vi "2 axis-Move.vi"(1 "error in (no error)":errorcluster, 2 "Deceleration":bool, 5 "RESET":bool, 6 "Accelaration":bool, 7 "B axis":i32, 8 "Stop":bool, 9 "A axis":i32, 10 "Comport":refnum<visa-resource-name>="COM4") -> (3 "A out":dbl, 4 "B out":dbl)   [LabVIEW 2023]
uses:
  <vilib>/Instr/_visa.llb/VISA Configure Serial Port (Instr).vi
  Holmarc/2 axis linear/GlobalValue.vi
panel:
  out "x-y 2":u32
  out "x-y":u32
  out "Process 3":u32
  out "Process 2":u32
  out "movement\ntime":u32
  out "First loop":u32
  # "COMPORT"
  # "To Move"
  # "Moved"
  # "Microns"
  # "Microns"
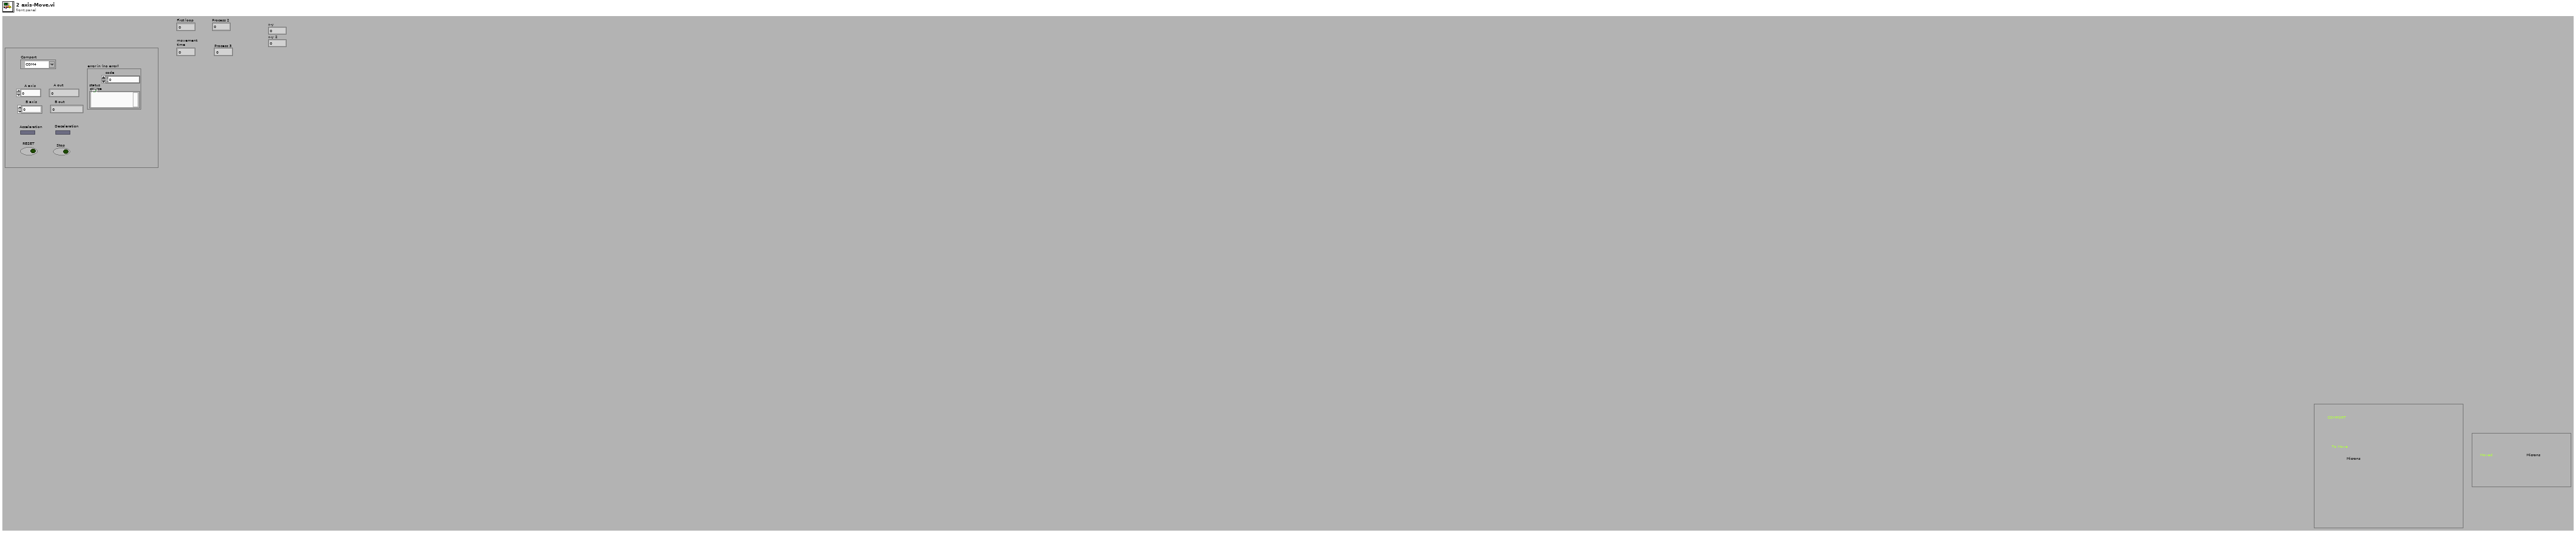
[diagram p1: front panel]
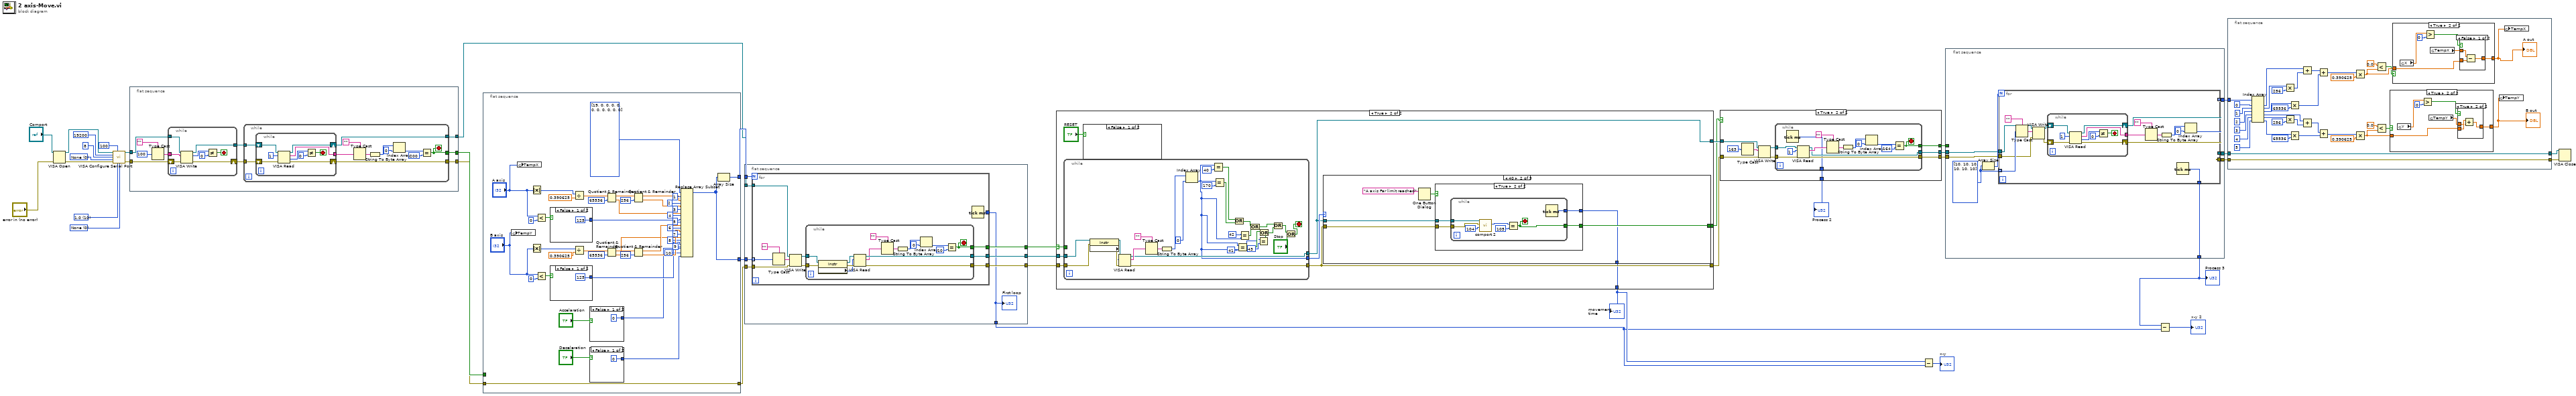
[diagram p0: block diagram]
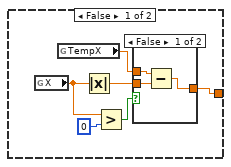
[diagram p2: hidden frame]
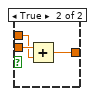
[diagram p3: hidden frame]
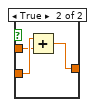
[diagram p4: hidden frame]
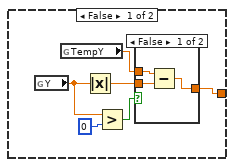
[diagram p5: hidden frame]
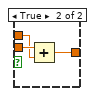
[diagram p6: hidden frame]
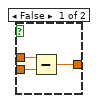
[diagram p7: hidden frame]
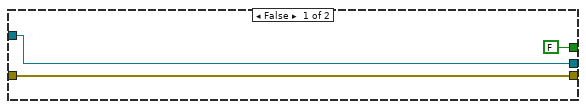
[diagram p8: hidden frame]
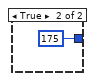
[diagram p9: hidden frame]
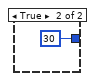
[diagram p10: hidden frame]
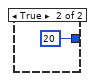
[diagram p11: hidden frame]
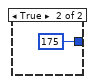
[diagram p12: hidden frame]
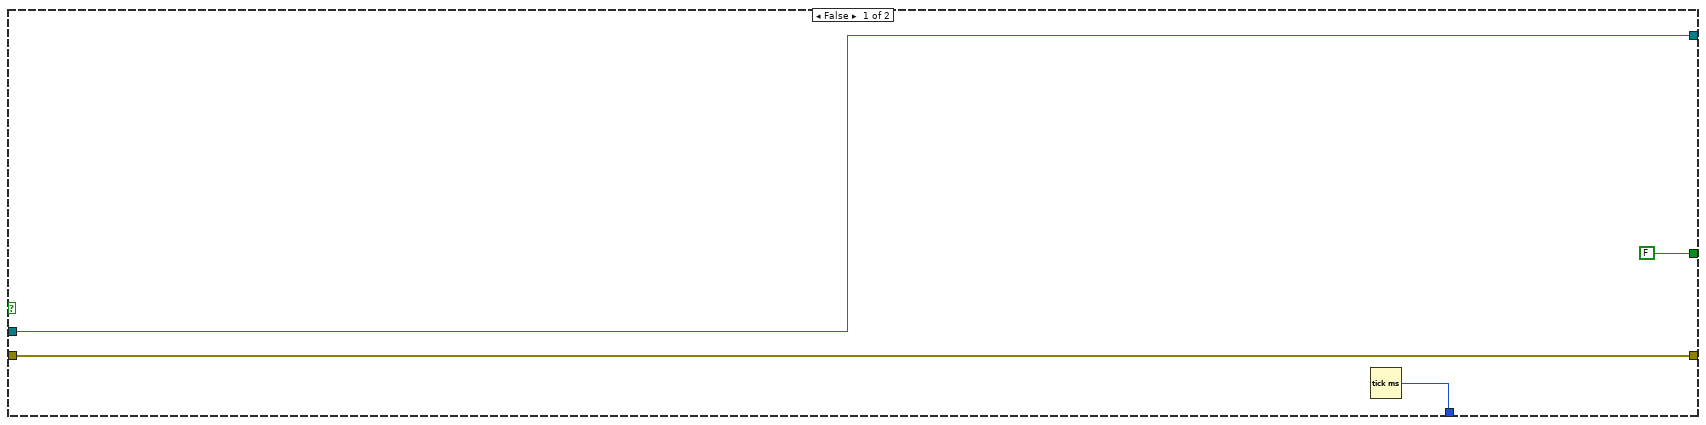
[diagram p13: hidden frame]
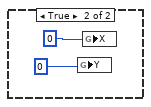
[diagram p14: hidden frame]
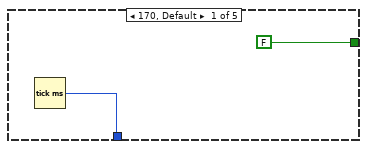
[diagram p15: hidden frame]
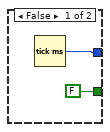
[diagram p16: hidden frame]
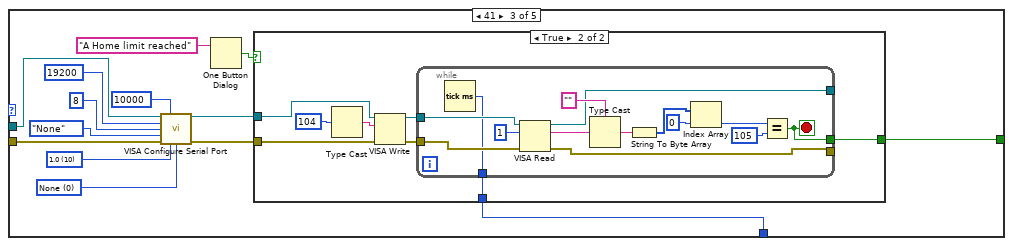
[diagram p17: hidden frame]
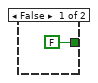
[diagram p18: hidden frame]
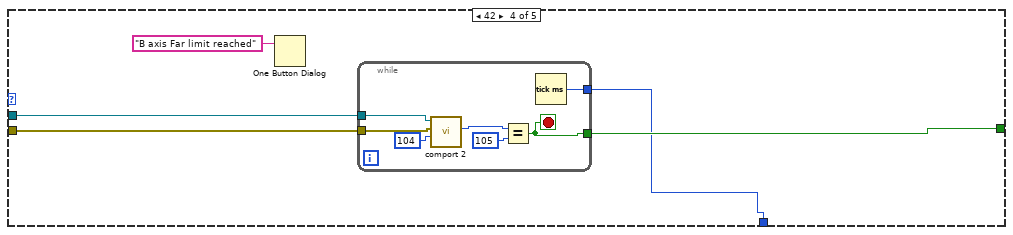
[diagram p19: hidden frame]
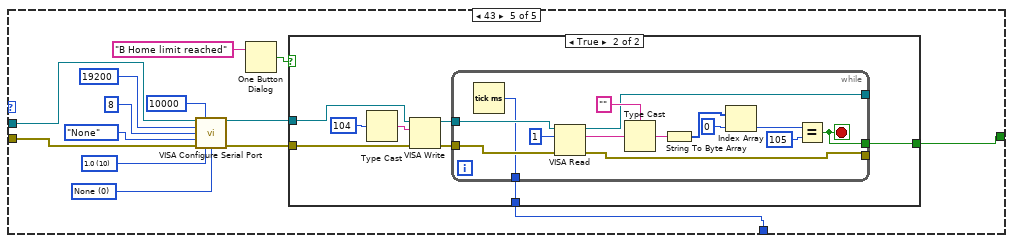
[diagram p20: hidden frame]
diagram:
  w33 = u16 0 items=["None"=0, "XON/XOFF"=1, "RTS/CTS"=2, "DTR/DSR"=4] ("flow control")
  w32 = u16 10 items=["1.0"=10, "1.5"=15, "2.0"=20] ("stop bits")
  w31 = u16 0 items=["None", "Odd", "Even", "Mark", "Space"] ("parity")
  n1 = VISA Open(error in (no error)="error in (no error)", VISA resource name="Comport") -> (VISA resource name=w36:refnum<visa-resource-name>, error out=w37:errorcluster)  [unwired: 3 in]
  n2 = call-poly "VISA Configure Serial Port"("VISA resource name"=w36, "timeout (10sec)"=u32 100, "baud rate (9600)"=u32 19200 ("baud rate"), "data bits (8)"=u16 8 ("data bits"), "parity (0:none)"=w31, "error in (no error)"=w37, "stop bits (10: 1 bit)"=w32, "flow control (0:none)"=w33) -> ("VISA resource name out"=w28:refnum<visa-resource-name>, "error out"=w27:errorcluster)  [unwired: 1 in, 5 out]
  n3 = flat-sequence {
    tunnel: w28 -> [w48]
    tunnel: w27 -> [w47]
    tunnel: [w46] -> w25
    tunnel: [w45] -> w12
    tunnel: [w39] -> w13
    frame #0 {
      n4 = Type Cast(type="", x=u8 100) -> (*(type *) &x=w43:string)
      n5 = while {
        tunnel: w43 -> [w56]
        shift-right: [w52] -> w40
        shift-left: w47 -> [w54]
        tunnel: w48 -> [w55]
        tunnel: [w53] -> w41
        stop <- w49 stop-if-true
        n6 = VISA Write(VISA resource name=w55, write buffer=w56, error in (no error)=w54) -> (VISA resource name out=w53:refnum<visa-resource-name>, return count=w51:u32, error out=w52:errorcluster)
        n7 = Not Equal?(x=w51, y=u32 0) -> (x != y?=w49:bool)
      }
      n8 = while {
        tunnel: w40 -> [w67]
        tunnel: [w65] -> w45
        tunnel: w41 -> [w68]
        tunnel: [w66] -> w46
        tunnel: [w60] -> w39
        stop <- w60 stop-if-true
        n9 = while {
          tunnel: [w72] -> w59
          shift-right: [w75] -> w66
          shift-left: w68 -> [w77]
          shift-right: [w74] -> w65
          shift-left: w67 -> [w76]
          stop <- w69 stop-if-true
          n10 = VISA Read(VISA resource name=w77, byte count=u32 1, error in (no error)=w76) -> (VISA resource name out=w75:refnum<visa-resource-name>, read buffer=w72:string, return count=w70:u32, error out=w74:errorcluster)
          n11 = Not Equal?(x=w70, y=u32 0) -> (x != y?=w69:bool)
        }
        n12 = Type Cast(type="", x=w59) -> (*(type *) &x=w57:string)
        n13 = String To Byte Array(string=w57) -> (unsigned byte array=w64:u8[])
        n14 = Index Array(array=w64, index=0) -> (element=w62:u8)
        n15 = Equal?(x=w62, y=u8 200) -> (x = y?=w60:bool)
      }
    }
  }
  n16 = flat-sequence {
    tunnel: [w116] -> w26
    tunnel: [w78] -> w24
    tunnel: w13 -> [_]
    tunnel: w12 -> [w113]
    tunnel: [w113] -> w11
    frame #0 {
      n17 = global write "GlobalValue.vi" "TempY"("B axis") -> ()
      n18 = global write "GlobalValue.vi" "TempX"("A axis") -> ()
      n19 = Absolute Value(x="A axis") -> (abs(x)=w117:i32)
      n20 = Absolute Value(x="B axis") -> (abs(x)=w105:i32)
      n21 = Less?(x="A axis", y=0) -> (x < y?=w119:bool)
      n22 = Less?(x="B axis", y=0) -> (x < y?=w100:bool)
      n23 = case shown="False" w119 {
        tunnel: [u16 125 u16 175] -> w91
        frame False {
        }
        frame True {
        }
      }
      n24 = case shown="False" w100 {
        tunnel: [u16 125 u16 175] -> w83
        frame False {
        }
        frame True {
        }
      }
      n25 = Divide(x=w117, y=0.390625) -> (x/y=w112:dbl)
      n26 = Divide(x=w105, y=0.390625) -> (x/y=w104:dbl)
      n27 = case shown="False" "Accelaration" {
        tunnel: [0 20] -> w81
        frame False {
        }
        frame True {
        }
      }
      n28 = case shown="False" "Deceleration" {
        tunnel: [0 30] -> w79
        frame False {
        }
        frame True {
        }
      }
      n29 = Quotient & Remainder(x=w112, y=65536) -> (x-y*floor(x/y)=w110:dbl, floor(x/y)=w94:dbl)
      n30 = Quotient & Remainder(x=w104, y=65536) -> (x-y*floor(x/y)=w102:dbl, floor(x/y)=w85:dbl)
      n31 = Quotient & Remainder(x=w110, y=256) -> (x-y*floor(x/y)=w97:dbl, floor(x/y)=w96:dbl)
      n32 = Quotient & Remainder(x=w102, y=256) -> (x-y*floor(x/y)=w89:dbl, floor(x/y)=w87:dbl)
      n33 = Replace Array Subset(array=u8[] [19, 0, 0, 0, 0, 0, 0, 0, 0, 0, 0], new element #1=w97, index #1=1 ("index"), new element #2=w96, index #2=2 ("index"), new element #3=w94, index #3=3 ("index"), new element #4=w91, index #4=4 ("index"), new element #5=w89, index #5=5 ("index"), new element #6=w87, index #6=6 ("index"), new element #7=w85, index #7=7 ("index"), new element #8=w83, index #8=8 ("index"), new element #9=w81, index #9=9 ("index"), new element #10=w79, index #10=10 ("index")) -> (w78:u8[])
      n34 = Array Size(array=w78) -> (size(s)=w116:i32)
    }
  }
  n35 = flat-sequence {
    tunnel: w26 -> [w137]
    tunnel: w25 -> [w136]
    tunnel: w11 -> [w135]
    tunnel: w24 -> [w134]
    tunnel: [w133] -> w23
    tunnel: [w132] -> w10
    tunnel: [w131] -> w22
    tunnel: [w130] -> w3
    frame #0 {
      n36 = for {
        N: w137 -> [_]
        tunnel: [w143] -> w131
        tunnel: w136 -> [w147]
        tunnel: [w145] -> w133
        tunnel: w135 -> [w146]
        tunnel: [w144] -> w132
        tunnel: w134 -> [w140] mode=indexing
        tunnel: [w138] -> w130
        n37 = Type Cast(type="", x=w140) -> (*(type *) &x=w139:string)
        n38 = VISA Write(VISA resource name=w147, write buffer=w139, error in (no error)=w146) -> (VISA resource name out=w142:refnum<visa-resource-name>, error out=w141:errorcluster)  [unwired: 1 out]
        n39 = while {
          tunnel: w141 -> [w152]
          tunnel: [w162] -> w144
          tunnel: w142 -> [w153]
          tunnel: [w163] -> w145
          tunnel: [w157] -> w143
          stop <- w157 stop-if-true
          n40 = property class="Instr"(reference=w153, error in=w152) -> (reference out=w151:refnum<visa-resource-name>, error out=w150:errorcluster, "Serial Settings:Number of Bytes at Serial Port"=w149:u32)
          n41 = VISA Read(VISA resource name=w151, byte count=w149, error in (no error)=w150) -> (VISA resource name out=w163:refnum<visa-resource-name>, read buffer=w156:string, error out=w162:errorcluster)  [unwired: 1 out]
          n42 = Type Cast(type="", x=w156) -> (*(type *) &x=w154:string)
          n43 = String To Byte Array(string=w154) -> (unsigned byte array=w161:u8[])
          n44 = Index Array(array=w161, index=0) -> (element=w159:u8)
          n45 = Equal?(x=w159, y=u8 10) -> (x = y?=w157:bool)
        }
        n46 = Tick Count (ms)() -> (millisecond timer value=w138:u32)
      }
      "First loop" <- w130
    }
  }
  n47 = case shown="True" w22 {
    selector: w22 -> [_ w169]
    tunnel: w23 -> [w167 w173]
    tunnel: w10 -> [w166 w175]
    tunnel: [w167 w172] -> w21
    tunnel: [w166 w171] -> w20
    tunnel: [FALSE w170] -> w7
    tunnel: [w164 w168] -> w5
    frame False {
      n48 = Tick Count (ms)() -> (millisecond timer value=w164:u32)
    }
    frame True {
      n49 = while {
        tunnel: w175 -> [w191]
        tunnel: [w195] -> w172
        tunnel: [w197] -> w171
        tunnel: [w177] -> w174
        tunnel: w173 -> [w192]
        tunnel: w169 -> [_]
        stop <- w178 stop-if-true
        n50 = property class="Instr"(reference=w192, error in=w191) -> (reference out=w190:refnum<visa-resource-name>, error out=w189:errorcluster, "Serial Settings:Number of Bytes at Serial Port"=w188:u32)
        n51 = VISA Read(VISA resource name=w190, byte count=w188, error in (no error)=w189) -> (VISA resource name out=w195:refnum<visa-resource-name>, read buffer=w204:string, error out=w197:errorcluster)  [unwired: 1 out]
        n52 = Type Cast(type="", x=w204) -> (*(type *) &x=w205:string)
        n53 = String To Byte Array(string=w205) -> (unsigned byte array=w203:u8[])
        n54 = Index Array(array=w203, index=0) -> (element=w177:u8)
        n55 = Equal?(x=w177, y=u8 40) -> (x = y?=w194:bool)
        n56 = Equal?(x=w177, y=u8 170) -> (x = y?=w196:bool)
        n57 = Or(x=w194, y=w196) -> (x .or. y?=w185:bool)
        n58 = Equal?(x=w177, y=u8 41) -> (x = y?=w183:bool)
        n59 = Equal?(x=u8 42 ("y"), y=w177) -> (x = y?=w184:bool)
        n60 = Or(x=w185, y=w184) -> (x .or. y?=w193:bool)
        n61 = Equal?(x=w177, y=u8 43) -> (x = y?=w182:bool)
        n62 = Or(x=w183, y=w182) -> (x .or. y?=w181:bool)
        n63 = Or(x=w193, y=w181) -> (x .or. y?=w180:bool)
        n64 = Or(x=w180, y="Stop") -> (x .or. y?=w178:bool)
      }
      n65 = case shown="False" "RESET" {
        frame False {
        }
        frame True {
          n66 = global write "GlobalValue.vi" "Y"(0) -> ()
          n67 = global write "GlobalValue.vi" "X"(0) -> ()
        }
      }
      n68 = case shown="40" w174 {
        tunnel: w172 -> [_ w212 w239 w269 w281]
        tunnel: w171 -> [_ w213 w236 w268 w280]
        tunnel: [FALSE w211 w240 w267 w279] -> w170
        tunnel: [w208 w210 w229 w266 w278] -> w168
        frame 170, Default {
          n69 = Tick Count (ms)() -> (millisecond timer value=w208:u32)
        }
        frame 40 {
          n70 = One Button Dialog(message="A axis Far limit reached") -> (true=w214:bool)  [unwired: 1 in]
          n71 = case shown="True" w214 {
            tunnel: w213 -> [_ w220]
            tunnel: w212 -> [_ w221]
            tunnel: [FALSE w219] -> w211
            tunnel: [w216 w218] -> w210
            frame False {
              n72 = Tick Count (ms)() -> (millisecond timer value=w216:u32)
            }
            frame True {
              n73 = while {
                tunnel: w221 -> [w228]
                tunnel: w220 -> [w227]
                tunnel: [w223] -> w219
                tunnel: [w222] -> w218
                stop <- w223 stop-if-true
                n74 = call "comport 2.vi"("x"=u8 104, "error in (no error)"=w227, "VISA resource name"=w228) -> ("Numeric"=w225:u8)  [unwired: 6 in, 2 out]
                n75 = Equal?(x=w225, y=u8 105) -> (x = y?=w223:bool)
                n76 = Tick Count (ms)() -> (millisecond timer value=w222:u32)
              }
            }
          }
        }
        frame 41 {
          w231 = u16 0 items=["None", "XON/XOFF", "RTS/CTS", "XON/XOFF & RTS/CTS", "DTR/DSR", "XON/XOFF & DTR/DSR"] ("flow control (0:none)")
          w232 = u16 10 items=["1.0"=10, "1.5"=15, "2.0"=20] ("stop bits (10: 1 bit)")
          n77 = call-poly "VISA Configure Serial Port"("VISA resource name"=w239, "timeout (10sec)"=u32 10000, "baud rate (9600)"=u32 19200, "data bits (8)"=u16 8, "parity (0:none)"=enum16{"None", "Odd", "Even", "Mark", "Space"}."None", "error in (no error)"=w236, "stop bits (10: 1 bit)"=w232, "flow control (0:none)"=w231) -> ("VISA resource name out"=w238:refnum<visa-resource-name>, "error out"=w237:errorcluster)  [unwired: 6 in]
          n78 = One Button Dialog(message="A Home limit reached") -> (true=w241:bool)  [unwired: 1 in]
          n79 = case shown="True" w241 {
            tunnel: w238 -> [_ w248]
            tunnel: w237 -> [_ w247]
            tunnel: [FALSE w245] -> w240
            tunnel: [_ w244] -> w229
            frame False {
            }
            frame True {
              n80 = Type Cast(x=104) -> (*(type *) &x=w251:string)  [unwired: 1 in]
              n81 = VISA Write(VISA resource name=w248, write buffer=w251, error in (no error)=w247) -> (VISA resource name out=w249:refnum<visa-resource-name>, error out=w250:errorcluster)  [unwired: 1 out]
              n82 = while {
                tunnel: w250 -> [w265]
                tunnel: [w255] -> _
                tunnel: w249 -> [w264]
                tunnel: [w254] -> _
                tunnel: [w253] -> w245
                tunnel: [w252] -> w244
                stop <- w253 stop-if-true
                n83 = Tick Count (ms)() -> (millisecond timer value=w252:u32)
                n84 = VISA Read(VISA resource name=w264, byte count=u32 1, error in (no error)=w265) -> (VISA resource name out=w254:refnum<visa-resource-name>, read buffer=w256:string, error out=w255:errorcluster)  [unwired: 1 out]
                n85 = Type Cast(type="", x=w256) -> (*(type *) &x=w257:string)
                n86 = String To Byte Array(string=w257) -> (unsigned byte array=w261:u8[])
                n87 = Index Array(array=w261, index=0) -> (element=w258:u8)
                n88 = Equal?(x=w258, y=u8 105) -> (x = y?=w253:bool)
              }
            }
          }
        }
        frame 42 {
          n89 = One Button Dialog(message="B axis Far limit reached") -> ()  [unwired: 1 in, 1 out]
          n90 = while {
            tunnel: [w274] -> w267
            tunnel: w269 -> [w273]
            tunnel: w268 -> [w272]
            tunnel: [w271] -> w266
            stop <- w274 stop-if-true
            n91 = call "comport 2.vi"("x"=u8 104, "error in (no error)"=w272, "VISA resource name"=w273) -> ("Numeric"=w276:u8)  [unwired: 6 in, 2 out]
            n92 = Equal?(x=w276, y=u8 105) -> (x = y?=w274:bool)
            n93 = Tick Count (ms)() -> (millisecond timer value=w271:u32)
          }
        }
        frame 43 {
          w283 = u16 0 items=["None", "XON/XOFF", "RTS/CTS", "XON/XOFF & RTS/CTS", "DTR/DSR", "XON/XOFF & DTR/DSR"] ("flow control (0:none)")
          w284 = u16 10 items=["1.0"=10, "1.5"=15, "2.0"=20] ("stop bits (10: 1 bit)")
          n94 = call-poly "VISA Configure Serial Port"("VISA resource name"=w281, "timeout (10sec)"=u32 10000, "baud rate (9600)"=u32 19200, "data bits (8)"=u16 8, "parity (0:none)"=enum16{"None", "Odd", "Even", "Mark", "Space"}."None", "error in (no error)"=w280, "stop bits (10: 1 bit)"=w284, "flow control (0:none)"=w283) -> ("VISA resource name out"=w289:refnum<visa-resource-name>, "error out"=w288:errorcluster)  [unwired: 6 in]
          n95 = One Button Dialog(message="B Home limit reached") -> (true=w290:bool)  [unwired: 1 in]
          n96 = case shown="True" w290 {
            tunnel: w289 -> [_ w297]
            tunnel: w288 -> [_ w296]
            tunnel: [FALSE w294] -> w279
            tunnel: [_ w293] -> w278
            frame False {
            }
            frame True {
              n97 = Type Cast(x=104) -> (*(type *) &x=w300:string)  [unwired: 1 in]
              n98 = VISA Write(VISA resource name=w297, write buffer=w300, error in (no error)=w296) -> (VISA resource name out=w298:refnum<visa-resource-name>, error out=w299:errorcluster)  [unwired: 1 out]
              n99 = while {
                tunnel: w299 -> [w314]
                tunnel: [w304] -> _
                tunnel: w298 -> [w313]
                tunnel: [w303] -> _
                tunnel: [w302] -> w294
                tunnel: [w301] -> w293
                stop <- w302 stop-if-true
                n100 = Tick Count (ms)() -> (millisecond timer value=w301:u32)
                n101 = VISA Read(VISA resource name=w313, byte count=u32 1, error in (no error)=w314) -> (VISA resource name out=w303:refnum<visa-resource-name>, read buffer=w305:string, error out=w304:errorcluster)  [unwired: 1 out]
                n102 = Type Cast(type="", x=w305) -> (*(type *) &x=w306:string)
                n103 = String To Byte Array(string=w306) -> (unsigned byte array=w310:u8[])
                n104 = Index Array(array=w310, index=0) -> (element=w307:u8)
                n105 = Equal?(x=w307, y=u8 105) -> (x = y?=w302:bool)
              }
            }
          }
        }
      }
    }
  }
  "movement\ntime" <- w5
  n106 = case shown="True" w7 {
    tunnel: w21 -> [w317 w324]
    tunnel: w20 -> [w316 w323]
    tunnel: [FALSE w322] -> w14
    tunnel: [w317 w320] -> w19
    tunnel: [w316 w321] -> w18
    tunnel: [_ w318] -> w6
    frame False {
    }
    frame True {
      n107 = Type Cast(x=163) -> (*(type *) &x=w327:string)  [unwired: 1 in]
      n108 = VISA Write(VISA resource name=w324, write buffer=w327, error in (no error)=w323) -> (VISA resource name out=w325:refnum<visa-resource-name>, error out=w326:errorcluster)  [unwired: 1 out]
      n109 = while {
        tunnel: w326 -> [w341]
        tunnel: [w331] -> w321
        tunnel: w325 -> [w340]
        tunnel: [w330] -> w322
        tunnel: [w329] -> w320
        tunnel: [w328] -> w318
        stop <- w330 stop-if-true
        n110 = Tick Count (ms)() -> (millisecond timer value=w328:u32)
        n111 = VISA Read(VISA resource name=w340, byte count=u32 1, error in (no error)=w341) -> (VISA resource name out=w329:refnum<visa-resource-name>, read buffer=w332:string, error out=w331:errorcluster)  [unwired: 1 out]
        n112 = Type Cast(type="", x=w332) -> (*(type *) &x=w333:string)
        n113 = String To Byte Array(string=w333) -> (unsigned byte array=w337:u8[])
        n114 = Index Array(array=w337, index=0) -> (element=w334:u8)
        n115 = Equal?(x=w334, y=u8 164) -> (x = y?=w330:bool)
      }
    }
  }
  "Process 2" <- w6
  n116 = Subtract(x=w5, y=w3) -> (x-y=→"x-y":u32)
  n117 = flat-sequence {
    tunnel: w18 -> [w348]
    tunnel: [w346] -> w16
    tunnel: [w347] -> w17
    tunnel: w19 -> [w345]
    tunnel: [w344] -> w15
    tunnel: w14 -> [_]
    tunnel: [w342] -> w2
    frame #0 {
      w343 = u8[] [10, 10, 10, 10, 10, 10]
      n118 = Array Size(array=w343) -> (size(s)=w349:i32)
      n119 = for {
        N: w349 -> [_]
        tunnel: w348 -> [w353]
        tunnel: [w360] -> w347
        tunnel: w345 -> [w354]
        tunnel: [w359] -> w346
        tunnel: [w358] -> w344 mode=indexing
        tunnel: w343 -> [w355] mode=indexing
        tunnel: [w350] -> w342
        n120 = Type Cast(type="", x=w355) -> (*(type *) &x=w356:string)
        n121 = VISA Write(VISA resource name=w354, write buffer=w356, error in (no error)=w353) -> (VISA resource name out=w352:refnum<visa-resource-name>, error out=w351:errorcluster)  [unwired: 1 out]
        n122 = while {
          tunnel: [w369] -> w363
          shift-right: [w372] -> w360
          shift-left: w352 -> [w374]
          shift-right: [w371] -> w359
          shift-left: w351 -> [w373]
          stop <- w366 stop-if-true
          n123 = VISA Read(VISA resource name=w374, byte count=u32 1, error in (no error)=w373) -> (VISA resource name out=w372:refnum<visa-resource-name>, read buffer=w369:string, return count=w367:u32, error out=w371:errorcluster)
          n124 = Not Equal?(x=w367, y=u32 0) -> (x != y?=w366:bool)
        }
        n125 = Type Cast(type="", x=w363) -> (*(type *) &x=w361:string)
        n126 = String To Byte Array(string=w361) -> (unsigned byte array=w365:u8[])
        n127 = Tick Count (ms)() -> (millisecond timer value=w350:u32)
        n128 = Index Array(array=w365, index=0) -> (element=w358:u8)
      }
    }
  }
  n129 = Subtract(x=w2, y=w3) -> (x-y=→"x-y 2":u32)
  n130 = flat-sequence {
    tunnel: w17 -> [w380]
    tunnel: w16 -> [w379]
    tunnel: w15 -> [w411]
    tunnel: [w380] -> w9
    tunnel: [w379] -> w8
    frame #0 {
      n131 = Index Array(array=w411, index #1=0 ("index"), index #2=1 ("index"), index #3=2 ("index"), index #4=3 ("index"), index #5=4 ("index"), index #6=5 ("index")) -> (element #1=w401:u8, element #2=w388:u8, element #3=w387:u8, element #4=w383:u8, element #5=w382:u8, element #6=w381:u8)
      n132 = Multiply(x=w388, y=u16 256) -> (x*y=w407:u16)
      n133 = Multiply(x=w382, y=u16 256) -> (x*y=w397:u16)
      n134 = Multiply(x=w387, y=u32 65536) -> (x*y=w406:u32)
      n135 = Multiply(x=w381, y=u32 65536) -> (x*y=w396:u32)
      n136 = Add(x=w401, y=w407) -> (x+y=w405:u16)
      n137 = Add(x=w383, y=w397) -> (x+y=w395:u16)
      n138 = Add(x=w405, y=w406) -> (x+y=w403:u32)
      n139 = Add(x=w395, y=w396) -> (x+y=w391:u32)
      n140 = Multiply(x=w403, y=0.390625) -> (x*y=w378:dbl)
      n141 = Multiply(x=w391, y=0.390625) -> (x*y=w392:dbl)
      n142 = Less?(x=0.0, y=w378) -> (x < y?=w375:bool)
      n143 = Less?(x=0.0, y=w392) -> (x < y?=w393:bool)
      n144 = case shown="True" w393 {
        tunnel: w392 -> [_ w448]
        tunnel: [w438 w450] -> w376
        frame False {
          n145 = global read "GlobalValue.vi" "Y"() -> (w437:dbl)
          n146 = global read "GlobalValue.vi" "TempY"() -> (w439:dbl)
          n147 = Absolute Value(x=w437) -> (abs(x)=w436:dbl)
          n148 = Greater?(x=w437, y=0) -> (0:w440:bool)
          n149 = case shown="False" w440 {
            tunnel: w436 -> [w443 w447]
            tunnel: w439 -> [w444 w446]
            tunnel: [w442 w445] -> w438
            frame False {
              n150 = Subtract(x=w444, y=w443) -> (x-y=w442:dbl)
            }
            frame True {
              n151 = Add(x=w447, y=w446) -> (x+y=w445:dbl)
            }
          }
        }
        frame True {
          n152 = global read "GlobalValue.vi" "Y"() -> (w449:dbl)
          n153 = Greater?(x=w449, y=0) -> (0:w452:bool)
          n154 = global read "GlobalValue.vi" "TempY"() -> (w451:dbl)
          n155 = case shown="True" w452 {
            tunnel: w448 -> [w455 w459]
            tunnel: w451 -> [w456 w458]
            tunnel: [w454 w457] -> w450
            frame False {
              n156 = Subtract(x=w456, y=w455) -> (x-y=w454:dbl)
            }
            frame True {
              n157 = Add(x=w459, y=w458) -> (x+y=w457:dbl)
            }
          }
        }
      }
      "B out" <- w376
      n158 = case shown="True" w375 {
        tunnel: w378 -> [_ w424]
        tunnel: [w414 w426] -> w377
        frame False {
          n159 = global read "GlobalValue.vi" "X"() -> (w413:dbl)
          n160 = global read "GlobalValue.vi" "TempX"() -> (w415:dbl)
          n161 = Absolute Value(x=w413) -> (abs(x)=w412:dbl)
          n162 = Greater?(x=w413, y=0) -> (0:w416:bool)
          n163 = case shown="False" w416 {
            tunnel: w412 -> [w419 w423]
            tunnel: w415 -> [w420 w422]
            tunnel: [w418 w421] -> w414
            frame False {
              n164 = Subtract(x=w420, y=w419) -> (x-y=w418:dbl)
            }
            frame True {
              n165 = Add(x=w423, y=w422) -> (x+y=w421:dbl)
            }
          }
        }
        frame True {
          n166 = global read "GlobalValue.vi" "X"() -> (w425:dbl)
          n167 = Greater?(x=w425, y=0) -> (0:w428:bool)
          n168 = global read "GlobalValue.vi" "TempX"() -> (w427:dbl)
          n169 = case shown="False" w428 {
            tunnel: w424 -> [w431 w435]
            tunnel: w427 -> [w432 w434]
            tunnel: [w430 w433] -> w426
            frame False {
              n170 = Subtract(x=w432, y=w431) -> (x-y=w430:dbl)
            }
            frame True {
              n171 = Add(x=w435, y=w434) -> (x+y=w433:dbl)
            }
          }
        }
      }
      "A out" <- w377
      n172 = global write "GlobalValue.vi" "TempY"(w376) -> ()
      n173 = global write "GlobalValue.vi" "TempX"(w377) -> ()
    }
  }
  n174 = VISA Close(VISA resource name=w9, error in (no error)=w8) -> ()  [unwired: 1 out]
  "Process 3" <- w2
